vi "UDP - Data Test (SubVI).vi"(8 "error in":errorcluster, 11 "data in":string) -> (0 "error out":errorcluster, 3 "Data Test":T1, 4 "Success":bool)   [LabVIEW 2019]
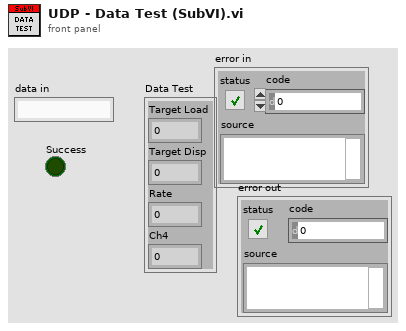
[diagram p1: front panel]
types:
  T1 = cluster{"Target Load":sgl, "Target Disp":sgl, "Rate":sgl, "Ch4":sgl}
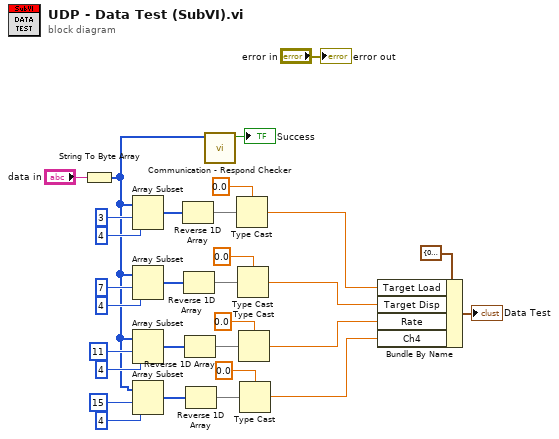
[diagram p0: block diagram]
diagram:
  n1 = String To Byte Array(string="data in") -> (unsigned byte array=w1:u8[])
  n2 = Array Subset(array=w1, index=3, length=4) -> (w21:u8[])
  n3 = Array Subset(array=w1, index=7, length=4) -> (w7:u8[])
  n4 = Array Subset(array=w1, index=11, length=4) -> (w6:u8[])
  n5 = Array Subset(array=w1, index=15, length=4) -> (w5:u8[])
  n6 = Reverse 1D Array(array=w21) -> (reversed array=w20:u8[])
  n7 = Reverse 1D Array(array=w7) -> (reversed array=w13:u8[])
  n8 = Reverse 1D Array(array=w6) -> (reversed array=w10:u8[])
  n9 = Reverse 1D Array(array=w5) -> (reversed array=w9:u8[])
  n10 = call "Communication - Respond Checker.vi"("Read Data"=w1) -> ("Success"=→"Success":bool)  [unwired: 10 in]
  n11 = Type Cast(type=sgl 0.0, x=w20) -> (*(type *) &x=w26:sgl)
  n12 = Type Cast(type=sgl 0.0, x=w13) -> (*(type *) &x=w27:sgl)
  n13 = Type Cast(type=sgl 0.0, x=w10) -> (*(type *) &x=w28:sgl)
  n14 = Type Cast(type=sgl 0.0, x=w9) -> (*(type *) &x=w29:sgl)
  n15 = Bundle By Name(cluster=T1 {"Target Load"=0.0, "Target Disp"=0.0, "Rate"=0.0, "Ch4"=0.0}, "Target Load"=w26, "Target Disp"=w27, "Rate"=w28, "Ch4"=w29) -> (→"Data Test":T1)
  "error out" <- "error in"
